vi "Ejercicio1_Case.vi"() -> ()   [LabVIEW 2022 SP3]
panel:
  in  "B":dbl
  in  "A":dbl
  out "Resultado":dbl
  in  "Operación":bool
  in  "stop":bool
  # "A+B"
  # "A-B"
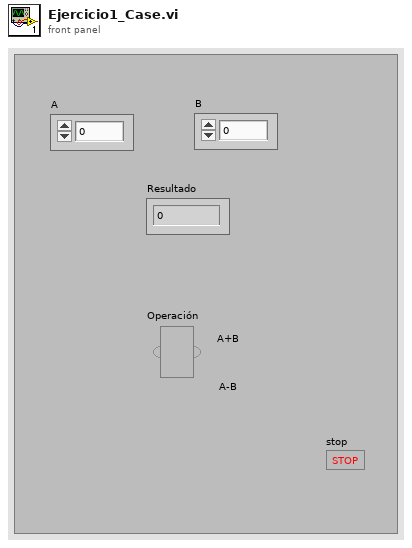
[diagram p1: front panel]
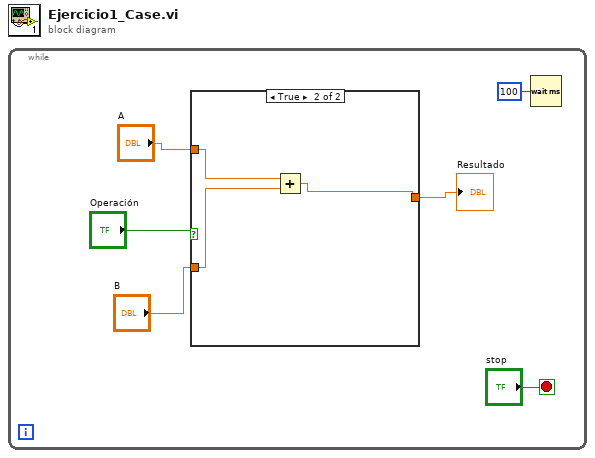
[diagram p0: block diagram]
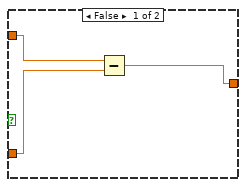
[diagram p2: hidden frame]
diagram:
  n1 = while {
    stop <- "stop" stop-if-true
    n2 = case shown="True" "Operación" {
      tunnel: [w7 w12] -> w3
      tunnel: "A" -> [w9 w11]
      tunnel: "B" -> [w8 w10]
      frame False {
        n3 = Subtract(x=w9, y=w8) -> (x-y=w7:dbl)
      }
      frame True {
        n4 = Add(x=w11, y=w10) -> (x+y=w12:dbl)
      }
    }
    "Resultado" <- w3
    n5 = Wait (ms)(milliseconds to wait=u32 100) -> ()  [unwired: 1 out]
  }
